vi "Destroy.vi"(8 "error in (no error)":errorcluster, 10 "Wait for Stop Timeout ms (-1)":i32=-1, 11 "API-Reference in":refnum<data-value>) -> (0 "error out":errorcluster, 1 "Timeout":bool, 3 "Final State":refnum<class "Actor.lvclass">)   [LabVIEW 2018, in "Scripting.lvlib" / "Actor.lvclass"]
uses:
  Actor.lvclass
  API-Data.ctl
  Did Stop.ctl
  Message-Enqueuer References.ctl
  Stop.ctl
  Launch.ctl
  Did Initialize.ctl
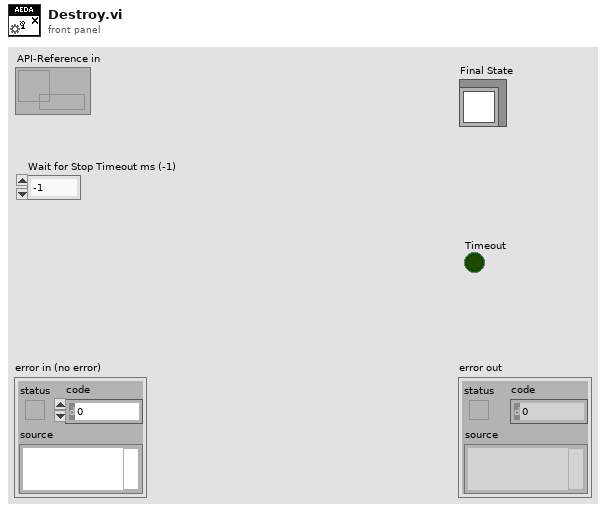
[diagram p1: front panel]
types:
  T1 = typedef "Scripting.lvlib/Actor.lvclass/API-Data.ctl" = cluster{"Launch":refnum<notifier>, "Did Stop Enqueuer":refnum<user-event>, "API":T2, "Did Stop Messages":refnum<event-registration>}
  T2 = typedef "Scripting.lvlib/Actor.lvclass/Message-Enqueuer References.ctl" = cluster{"Stop":refnum<user-event>, "Launch":refnum<user-event>, "Did Initialize":refnum<user-event>}
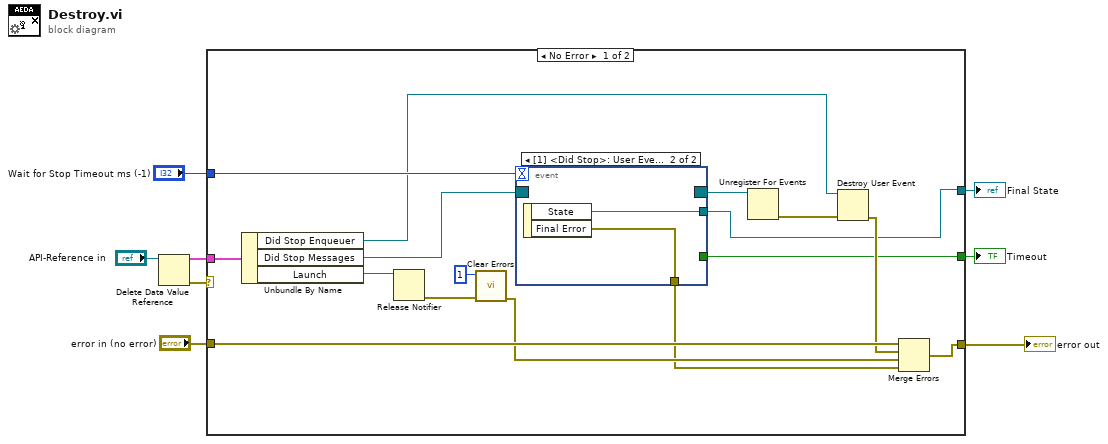
[diagram p0: block diagram]
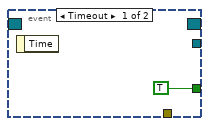
[diagram p2: hidden frame]
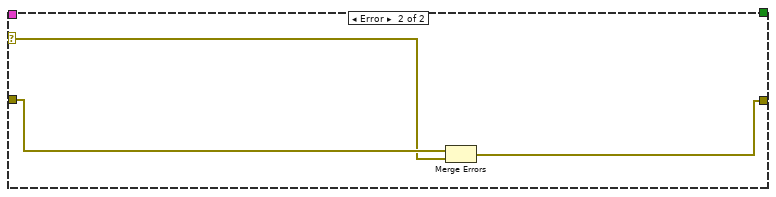
[diagram p3: hidden frame]
diagram:
  n1 = Delete Data Value Reference(data value reference="API-Reference in") -> (data value=w8:T1, error out=w4:errorcluster)  [unwired: 1 in]
  n2 = case shown="No Error" w4 {
    selector: w4 -> [_ w29]
    tunnel: w8 -> [w24 _]
    tunnel: "error in (no error)" -> [w23 w30]
    tunnel: "Wait for Stop Timeout ms (-1)" -> [w19 _]
    tunnel: [w18 w28] -> w5
    tunnel: [w10 _] -> w3
    tunnel: [w9 _] -> w2
    frame No Error {
      n3 = Unbundle By Name(w24) -> ("Did Stop Enqueuer"=w14:refnum<user-event>, "Did Stop Messages"=w20:refnum<event-registration>, "Launch"=w17:refnum<notifier>)
      n4 = Release Notifier(notifier=w17) -> (error out=w16:errorcluster)  [unwired: 2 in, 2 out]
      n5 = call <vilib>:"Clear Errors.vi"("error in (no error)"=w16, "specific error code to clear (0: all)"=1) -> ("error out"=w22:errorcluster)  [unwired: 4 in, 1 out]
      n6 = event shown="[1] <Did Stop>: User Event" {
        selector: w20 -> [_ _]
        dyn-events: [_ _] -> w12
        timeout: w19 -> [_ _]
        tunnel: [_ w27] -> w11
        tunnel: [TRUE _] -> w10
        tunnel: [_ w26] -> w9
        event Timeout {
          n7 = event-data() -> ()  [unwired: 1 in, 1 out]
        }
        event User Event {
          n8 = event-data() -> ("State"=w26:refnum<class "Actor.lvclass">, "Final Error"=w27:errorcluster)  [unwired: 1 in]
        }
      }
      n9 = Unregister For Events(event registration refnum=w12) -> (error out=w15:errorcluster)  [unwired: 1 in]
      n10 = Destroy User Event(user event=w14, error in=w15) -> (error out=w13:errorcluster)
      n11 = Merge Errors(w23, w13, w22, w11) -> (w18:errorcluster)
    }
    frame Error {
      n12 = Merge Errors(w30, w29) -> (w28:errorcluster)
    }
  }
  "error out" <- w5
  "Timeout" <- w3
  "Final State" <- w2
